vi "test Add-Find-Remove Port.vi"(8 "error in":errorcluster, 11 "TestCase in":refnum<class "Scripting.lvclass">=refnum) -> (0 "error out":errorcluster, 3 "TestCase out":refnum<class "Scripting.lvclass">)   [LabVIEW 2020, in "Scripting.lvclass"]
uses:
  Scripting.lvclass
  <vilib>/addons/_JKI Toolkits/VI Tester/TestCase.llb/TestCase.lvclass
  Scripting/AIM MIL-STD-1553 Scripting.lvlib
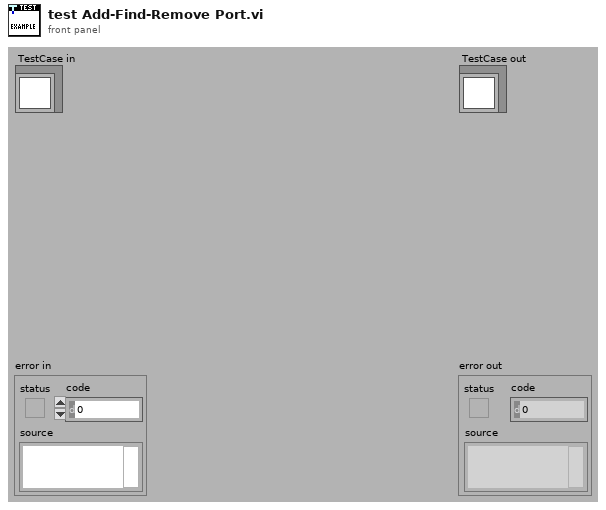
[diagram p1: front panel]
types:
  T1 = typedef "Custom Device API.lvlib/Custom Device Item Ref.ctl" = u64
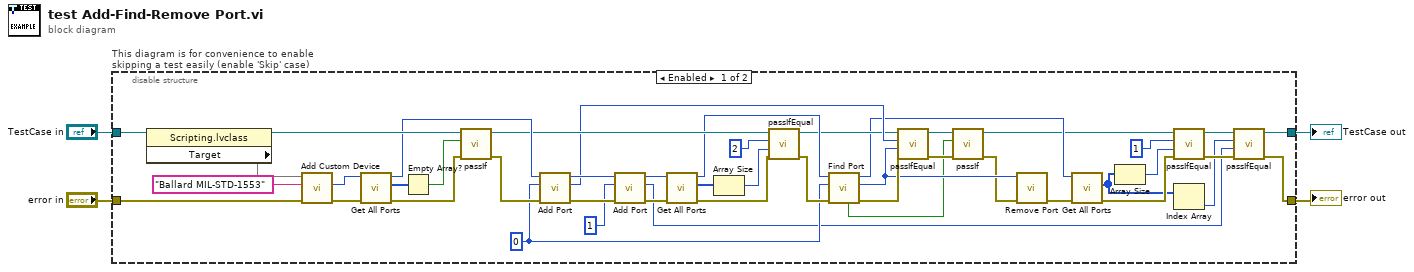
[diagram p0: block diagram]
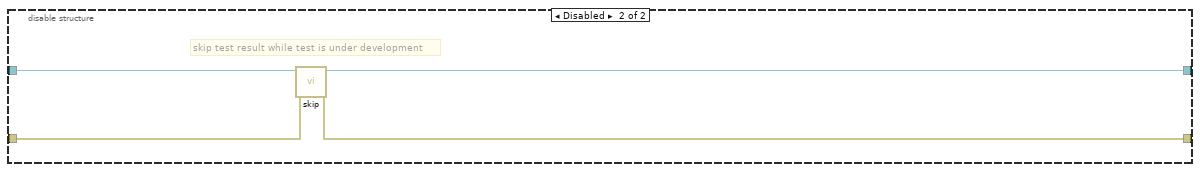
[diagram p2: hidden frame]
diagram:
  n1 = disable-structure "This diagram is for convenience to enable skipping a test easily (enable 'Skip' case)" shown="Enabled" {
    disable-tunnel: "TestCase in" -> [w48 w54]
    disable-tunnel: [w10 w52] -> w1
    disable-tunnel: [w14 w53] -> w3
    disable-tunnel: "error in" -> [w50 w51]
    frame Enabled {
      w26 = u16 0 ("port number")
      n2 = property class="Scripting.lvclass"(reference=w48) -> (reference out=w42:refnum<class "Scripting.lvclass">, "Target"=w47)  [unwired: 1 in, 1 out]
      n3 = call "Add Custom Device.vi"("error in"=w50, "name"="Ballard MIL-STD-1553", "target in"=w47) -> ("error out"=w46:errorcluster, "Ballard MIL-STD 1553 custom device"=w45:T1)  [unwired: 6 in, 1 out]
      n4 = call "Get All Ports.vi"("error in"=w46, "Ballard MIL-STD 1553 custom device in"=w45) -> ("error out"=w40:errorcluster, "ports"=w43:T1[], "Ballard MIL-STD 1553 custom device out"=w39:T1)  [unwired: 7 in]
      n5 = Empty Array?(array=w43) -> (empty?=w44:bool)
      n6 = call-dynamic "passIf.vi"("error in (no error)"=w40, "pass"=w44, "TestCase in"=w42) -> ("error out"=w41:errorcluster, "TestCase out"=w30:refnum<class "Scripting.lvclass">)  [unwired: 7 in]
      n7 = call "Add Port.vi"("error in"=w41, "port number"=w26, "Ballard MIL-STD 1553 custom device in"=w39) -> ("error out"=w38:errorcluster, "port"=w24:T1, "Ballard MIL-STD 1553 custom device out"=w37:T1)  [unwired: 6 in]
      n8 = call "Add Port.vi"("error in"=w38, "port number"=u16 1, "Ballard MIL-STD 1553 custom device in"=w37) -> ("error out"=w35:errorcluster, "port"=w12:T1, "Ballard MIL-STD 1553 custom device out"=w34:T1)  [unwired: 6 in]
      n9 = call "Get All Ports.vi"("error in"=w35, "Ballard MIL-STD 1553 custom device in"=w34) -> ("error out"=w29:errorcluster, "ports"=w33:T1[], "Ballard MIL-STD 1553 custom device out"=w27:T1)  [unwired: 7 in]
      n10 = Array Size(array=w33) -> (size(s)=w32:i32)
      n11 = call-dynamic "passIfEqual.vi"("error in (no error)"=w29, "y"=w32, "x"=2 ("size(s)"), "TestCase in"=w30) -> ("error out"=w28:errorcluster, "TestCase out"=w23:refnum<class "Scripting.lvclass">)  [unwired: 6 in]
      n12 = call "Find Port.vi"("error in"=w28, "port number"=w26, "Ballard MIL-STD 1553 custom device in"=w27) -> ("error out"=w25:errorcluster, "port"=w21:T1, "Ballard MIL-STD 1553 custom device out"=w22:T1, "found?"=w5:bool)  [unwired: 5 in]
      n13 = call-dynamic "passIfEqual.vi"("error in (no error)"=w25, "y"=w21, "x"=w24, "TestCase in"=w23) -> ("error out"=w9:errorcluster, "TestCase out"=w8:refnum<class "Scripting.lvclass">)  [unwired: 6 in]
      n14 = call-dynamic "passIf.vi"("error in (no error)"=w9, "pass"=w5, "TestCase in"=w8) -> ("error out"=w6:errorcluster, "TestCase out"=w7:refnum<class "Scripting.lvclass">)  [unwired: 7 in]
      n15 = call "Remove Port.vi"("error in"=w6, "port"=w21) -> ("error out"=w20:errorcluster)  [unwired: 9 in]
      n16 = call "Get All Ports.vi"("error in"=w20, "Ballard MIL-STD 1553 custom device in"=w22) -> ("error out"=w19:errorcluster, "ports"=w16:T1[])  [unwired: 7 in, 1 out]
      n17 = Array Size(array=w16) -> (size(s)=w18:i32)
      n18 = call-dynamic "passIfEqual.vi"("error in (no error)"=w19, "y"=w18, "x"=1 ("size(s)"), "TestCase in"=w7) -> ("error out"=w15:errorcluster, "TestCase out"=w11:refnum<class "Scripting.lvclass">)  [unwired: 6 in]
      n19 = Index Array(array=w16) -> (element=w13:T1)  [unwired: 1 in]
      n20 = call-dynamic "passIfEqual.vi"("error in (no error)"=w15, "y"=w12, "x"=w13, "TestCase in"=w11) -> ("error out"=w14:errorcluster, "TestCase out"=w10:refnum<class "Scripting.lvclass">)  [unwired: 6 in]
    }
    frame Disabled {
      # "skip test result while test is under development"
      n21 = call <vilib>:"skip.vi"("error in (no error)"=w51, "TestCase in"=w54) -> ("error out"=w53:errorcluster, "TestCase out"=w52:refnum<class "TestCase.lvclass">)  [unwired: 8 in]
    }
  }
  "error out" <- w3
  "TestCase out" <- w1
